vi "BKPrecision_PS_Shutdown.vi"(6 "Current Limit (0)":dbl min=0.0 max=6.0 format="%#.2g", 8 "error in (no error)":errorcluster, 9 "Output Voltage (0)":dbl min=0.0 max=31.0 format="%#.2f", 10 "Maximum Output Voltage (31)":dbl min=0.0 max=31.0 format="%#.2f", 11 "VISA resource name":refnum<visa-resource-name>) -> (0 "error out":errorcluster, 3 "VISA resource name out":refnum<visa-resource-name>)   [LabVIEW 2015]
uses:
  <instrlib>/BK Precision 178XB Series/BK Precision 178XB Series.lvlib
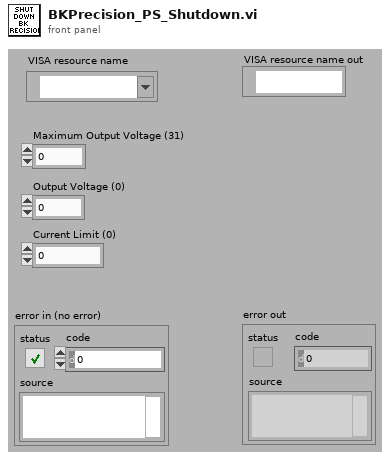
[diagram p1: front panel]
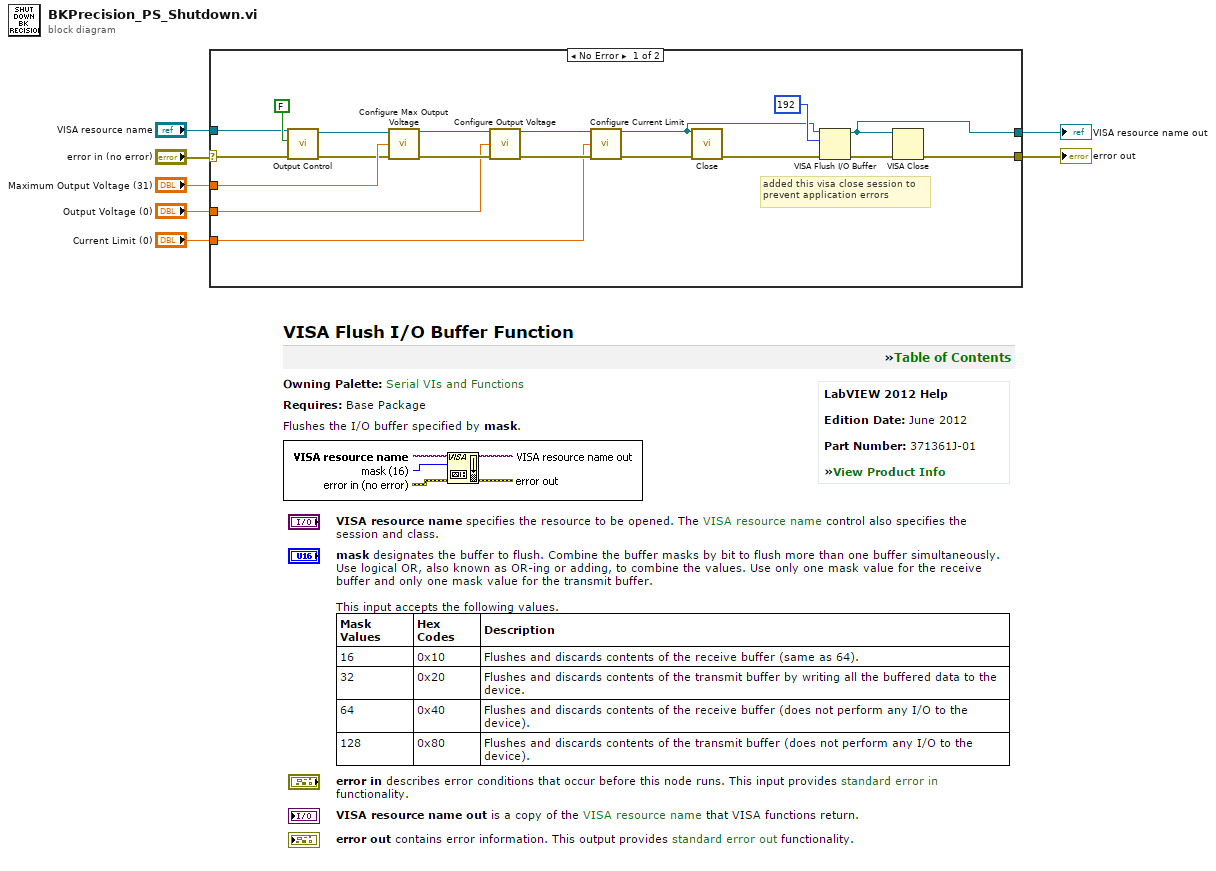
[diagram p0: block diagram]
diagram:
  n1 = case shown="No Error" "error in (no error)" {
    selector: "error in (no error)" -> [w12 w28]
    tunnel: "Maximum Output Voltage (31)" -> [w22 _]
    tunnel: "Output Voltage (0)" -> [w21 _]
    tunnel: "Current Limit (0)" -> [w20 _]
    tunnel: [w17 w28] -> w4
    tunnel: "VISA resource name" -> [w10 w27]
    tunnel: [w16 w27] -> w2
    frame No Error {
      # "added this visa close session to \nprevent application errors"
      n2 = call <instrlib>:"Output Control.vi"("error in (no error)"=w12, "Enable Output Terminals (F: Off)"=FALSE ("on"), "VISA resource name"=w10) -> ("error out"=w13:errorcluster, "VISA resource name out"=w9:refnum<visa-resource-name>)  [unwired: 7 in]
      n3 = call <instrlib>:"Configure Max Output Voltage.vi"("VISA resource name"=w9, "Maximum Output Voltage (18)"=w22, "error in (no error)"=w13) -> ("VISA resource name out"=w26:refnum<visa-resource-name>, "error out"=w23:errorcluster)  [unwired: 11 in]
      n4 = call <instrlib>:"Configure Output Voltage.vi"("VISA resource name"=w26, "Output Voltage (0)"=w21, "error in (no error)"=w23) -> ("VISA resource name out"=w25:refnum<visa-resource-name>, "error out"=w24:errorcluster)  [unwired: 11 in]
      n5 = call <instrlib>:"Configure Current Limit.vi"("VISA resource name"=w25, "Current Limit (0)"=w20, "error in (no error)"=w24) -> ("VISA resource name out"=w8:refnum<visa-resource-name>, "error out"=w15:errorcluster)  [unwired: 11 in]
      n6 = call <instrlib>:"Close.vi"("error in (no error)"=w15, "VISA resource name"=w8) -> ("error out"=w14:errorcluster)  [unwired: 9 in]
      n7 = VISA Flush I/O Buffer(VISA resource name=w8, mask (16)=u16 192, error in (no error)=w14) -> (VISA resource name out=w16:refnum<visa-resource-name>, error out=w19:errorcluster)
      n8 = VISA Close(VISA resource name=w16, error in (no error)=w19) -> (error out=w17:errorcluster)
    }
    frame Error {
    }
  }
  "error out" <- w4
  "VISA resource name out" <- w2
